vi "Power Accuracy Execute Measurement.vi"(0 "Plots":T11, 1 "Measurement Data In":T10[](array[typedef]), 2 "TestSetDef":T1={"General"={"ID"=0, "Model"="", "Dual Port?"=FALSE, "Options"="", "Options"={"E"=FALSE, "K"=FALSE, "H"=FALSE, "W"=FALSE, "F"=FALSE}, "Cal File"=path ""}, "Receiver"={"Fstart, MHz"=0.0, "Fstop MHz"=0.0, "Fstep MHz"=0.0, "IF, MHz"=0.0}, "RX Band"={"Fstart, MHz"=0.0, "Fstop MHz"=0.0}, "TX 1"={"Fstart, MHz"=0.0, "Fstop MHz"=0.0, "Pmax, dBm"=0.0, "Pstep, dB"=0.0}, "TX 2"={"Fstart, MHz"=0.0, "Fstop MHz"=0.0, "Pmax, dBm"=0.0, "Pstep, dB"=0.0}, "Low-side?"=TRUE}, 3 "Queue":refnum<queue>, 5 "Test Parameters":T2={"Stimulus"={"Power Start"=38, "Power Stop"=46, "Frequency Type"=enum."Band Edges", "Frequency Points"=[], "TX 1 Frequency (MHz)"={"Min"=0.0, "Max"=0.0}, "TX 2 Frequency (MHz)"={"Min"=0.0, "Max"=0.0}, "RX Frequency (MHz)"={"Min"=0.0, "Max"=0.0}, "Pad Model Number"="", "Pad Serial Number"="", "Pad Values"=[]}, "Measurement"={"DUT Port"=enum."Port 1", "Direction"=0}, "Display"={"Power"={"Min"=0, "Max"=0}, "Tolerance"={"Min"=0.0, "Max"=0.0}}, "Limit"={"Tolerance"=0.35}, "Calibration"={"Calibrated?"=FALSE}} {"Measurement"."Direction" items=["Reverse", "Forward", "Auxiliary"]}, 9 "Calculated Values":refnum<vi>, 11 "error in (no error)":errorcluster, 12 "Driver Refs In":T14, 13 "Measurements":refnum<vi>) -> (4 "Pass/Fail":bool[](array[boolean]), 6 "Test Parameters Out":T2={"Stimulus"={"Power Start"=38, "Power Stop"=46, "Frequency Type"=enum."Band Edges", "Frequency Points"=[], "TX 1 Frequency (MHz)"={"Min"=0.0, "Max"=0.0}, "TX 2 Frequency (MHz)"={"Min"=0.0, "Max"=0.0}, "RX Frequency (MHz)"={"Min"=0.0, "Max"=0.0}, "Pad Model Number"="", "Pad Serial Number"="", "Pad Values"=[]}, "Measurement"={"DUT Port"=enum."Port 1", "Direction"=0}, "Display"={"Power"={"Min"=0, "Max"=0}, "Tolerance"={"Min"=0.0, "Max"=0.0}}, "Limit"={"Tolerance"=0.35}, "Calibration"={"Calibrated?"=FALSE}} {"Measurement"."Direction" items=["Reverse", "Forward", "Auxiliary"]}, 10 "Measurement Data Out":T10[](array[typedef]), 14 "Driver Refs Out":T14, 15 "error out":errorcluster)   [LabVIEW 2011]
uses:
  TypeDefs/Power Accuracy Test Parameters.ctl
  TypeDefs/Power Accuracy Stimulus Parameters.ctl
  TypeDefs/Power Accuracy Measurement Parameters.ctl
  BPIMCore EXT/HW IO/DUTport.ctl
  BPIMCore EXT/HW IO/MeasMode.ctl
  TypeDefs/Power Accuracy Display Parameters.ctl
  TypeDefs/Power Accuracy Limit Parameters.ctl
  TypeDefs/Power Accuracy Calibration State.ctl
  drivers/PIM/PIM Driver Ref.ctl
  drivers/PWM/PWM Driver Ref.ctl
  TypeDefs/Power Accuracy Measurement Data.ctl
  TypeDefs/Power Accuracy Queue Cluster.ctl
  BPIMCore EXT/HW IO/Test Set Definition.ctl
  drivers/PIM/PIM Command.ctl
  drivers/PWM/PWM Parameters.ctl
  drivers/PWM/PWM Command.ctl
  Summitek EXT/Miscellaneous/OGAB Version.ctl
  <vilib>/Analysis/NI_AALBase.lvlib
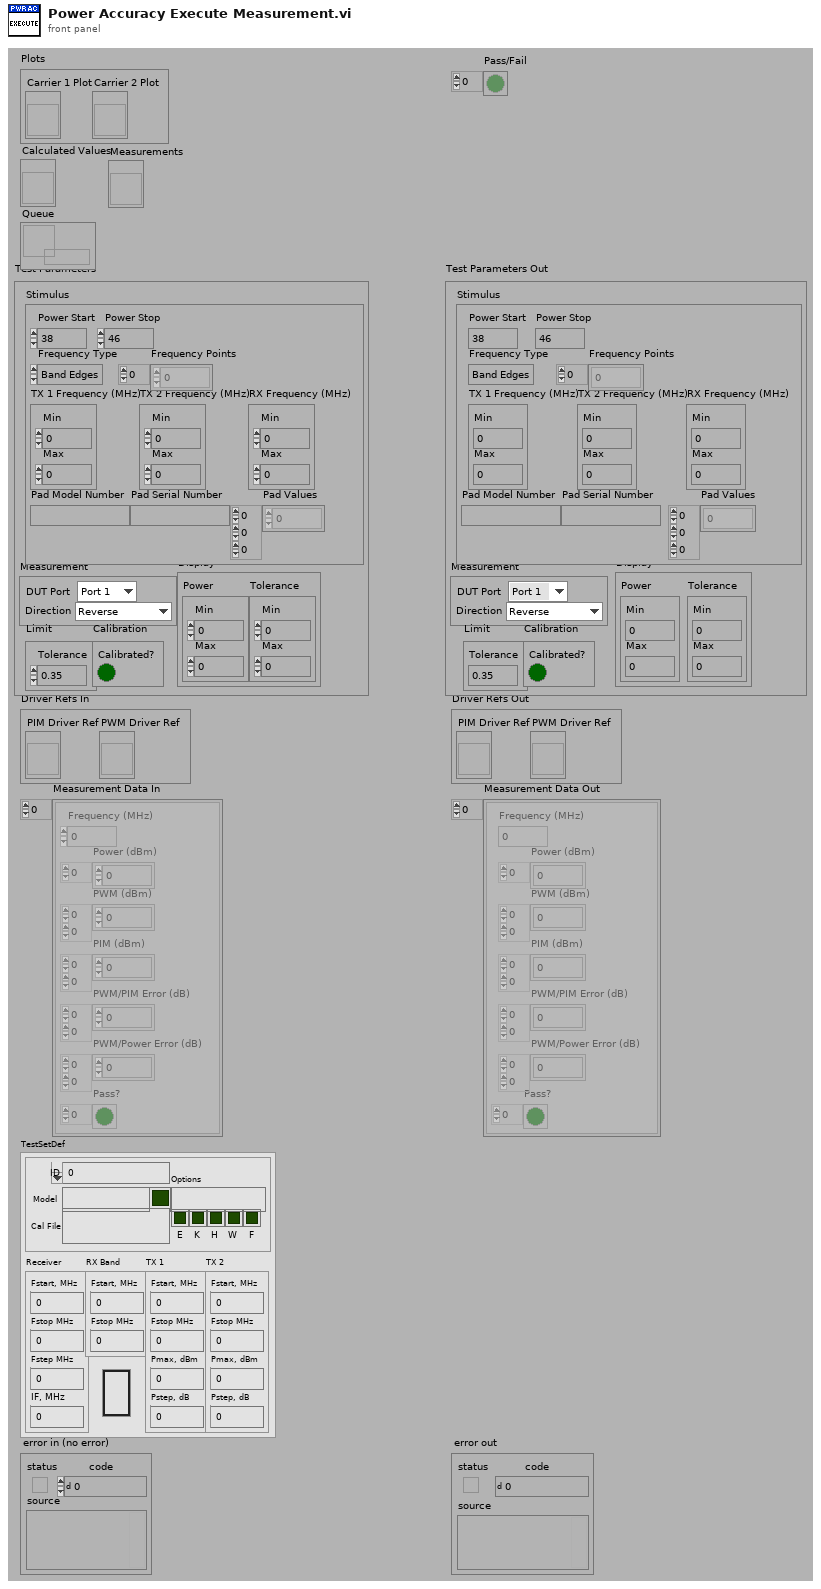
[diagram p1: front panel]
types:
  T1 = typedef "Test Set Definition.ctl" = cluster{"General":cluster{"ID":u32, "Model":string, "Dual Port?":bool, "Options":string, "Options":cluster{"E":bool, "K":bool, "H":bool, "W":bool, "F":bool}, "Cal File":path}, "Receiver":cluster{"Fstart, MHz":dbl, "Fstop MHz":dbl, "Fstep MHz":dbl, "IF, MHz":dbl}, "RX Band":cluster{"Fstart, MHz":dbl, "Fstop MHz":dbl}, "TX 1":cluster{"Fstart, MHz":dbl, "Fstop MHz":dbl, "Pmax, dBm":dbl, "Pstep, dB":dbl}, "TX 2":cluster{"Fstart, MHz":dbl, "Fstop MHz":dbl, "Pmax, dBm":dbl, "Pstep, dB":dbl}, "Low-side?":bool}
  T2 = typedef "Power Accuracy Test Parameters.ctl" = cluster{"Stimulus":T3, "Measurement":T4, "Display":T7, "Limit":T8, "Calibration":T9}
  T3 = typedef "Power Accuracy Stimulus Parameters.ctl" = cluster{"Power Start":i32, "Power Stop":i32, "Frequency Type":enum16{"Band Edges", "Custom"}, "Frequency Points":dbl[], "TX 1 Frequency (MHz)":cluster{"Min":dbl, "Max":dbl}, "TX 2 Frequency (MHz)":cluster{"Min":dbl, "Max":dbl}, "RX Frequency (MHz)":cluster{"Min":dbl, "Max":dbl}, "Pad Model Number":string, "Pad Serial Number":string, "Pad Values":dbl[][][]}
  T4 = typedef "Power Accuracy Measurement Parameters.ctl" = cluster{"DUT Port":T5, "Direction":T6}
  T5 = typedef "DUTport.ctl" = enum16{"Port 1", "Port 2"}
  T6 = typedef "MeasMode.ctl" = u16
  T7 = typedef "Power Accuracy Display Parameters.ctl" = cluster{"Power":cluster{"Min":i32, "Max":i32}, "Tolerance":cluster{"Min":dbl, "Max":dbl}}
  T8 = typedef "Power Accuracy Limit Parameters.ctl" = cluster{"Tolerance":dbl}
  T9 = typedef "Power Accuracy Calibration State.ctl" = cluster{"Calibrated?":bool}
  T10 = typedef "Power Accuracy Measurement Data.ctl" = cluster{"Frequency (MHz)":dbl, "Power (dBm)":i32[], "PWM (dBm)":dbl[][], "PIM (dBm)":dbl[][], "PWM/PIM Error (dB)":dbl[][], "PWM/Power Error (dB)":dbl[][], "Pass?":bool[]}
  T11 = cluster{"Carrier 1 Plot":refnum<vi>, "Carrier 2 Plot":refnum<vi>}
  T12 = typedef "PIM Driver Ref.ctl" = refnum<vi>
  T13 = typedef "PWM Driver Ref.ctl" = refnum<vi>
  T14 = cluster{"PIM Driver Ref":T12, "PWM Driver Ref":T13}
  T15 = typedef "PIM Stimulus.ctl" = cluster{"Carrier Frequencies":cluster{"C1 Freq, MHz":dbl, "C2 Freq, MHz":dbl}, "Carrier Powers":cluster{"C1 Power,dBm":dbl, "C2 Power, dBm":dbl}, "Measurement Parameters":T16, "Measurement Setup":cluster{"Meas Type":enum32{"Time", "Frequency"}, "TXStep":T20}}
  T16 = typedef "PIM Cmd Params.ctl" = cluster{"IM Order":T17, "Averaging":T18, "Direction":T6, "Enable ALC?":bool, "Enable SingleIM?":bool, "Display Units":T19, "VA Hold?":bool, "DUT PORT":T5}
  T17 = typedef "IMOrder.ctl" = u8
  T18 = typedef "HW Averaging.ctl" = u16
  T19 = typedef "display_unit_format.ctl" = enum16{"dBm", "dBc"}
  T20 = typedef "PIM Sweep Step Size.ctl" = u16
  T21 = typedef "PIM Command.ctl" = enum16{"LOAD", "KEEP ALIVE", "VALIDATE", "INITIALIZE", "PRESET", "GET CALIBRATION", "SET STIMULUS", "TOGGLE TX POWER", "SET TX ON", "SET TX OFF", "MEASURE", "UNLOAD"}
  T22 = typedef "PWM Parameters.ctl" = cluster{"Zero":bool, "Blank Screen":bool, "Offset":bool, "Offset Value":dbl, "Frequency (MHz)":dbl}
  T23 = typedef "PWM Command.ctl" = enum16{"LOAD", "INITIALIZE", "PRESET", "GET STIMULUS", "SET STIMULUS", "MEASURE", "RELEASE", "UNLOAD", "GET CALIBRATION", "CALIBRATE"}
  T24 = typedef "OGAB Version.ctl" = cluster{"Version":string, "Build Number":u32, "Build Date/Time":dbl}
  T25 = typedef "Power Accuracy Queue Cluster.ctl" = cluster{"Command":string, "Test Parameters":T2}
  T26 = typedef "PIM Results.ctl" = cluster{"TxFreqs":dbl[], "TxPower":dbl[], "TxOn":bool[], "IMPower(s)":dbl[], "IMFreq(s)":dbl[], "Tx Stat":cluster{"CheckTx 1":bool, "Unlev Tx 1":bool, "Sql Tx 1":bool, "CheckTx 2":bool, "Unlev Tx 2":bool, "Sql Tx 2":bool}, "IM Overload":bool, "IMPower_dBc(s)":dbl[]}
  T27 = typedef "PWM Measurement.ctl" = dbl
  T28 = cluster{"duplicate driver ref":T12, "PWM Driver Ref":T13}
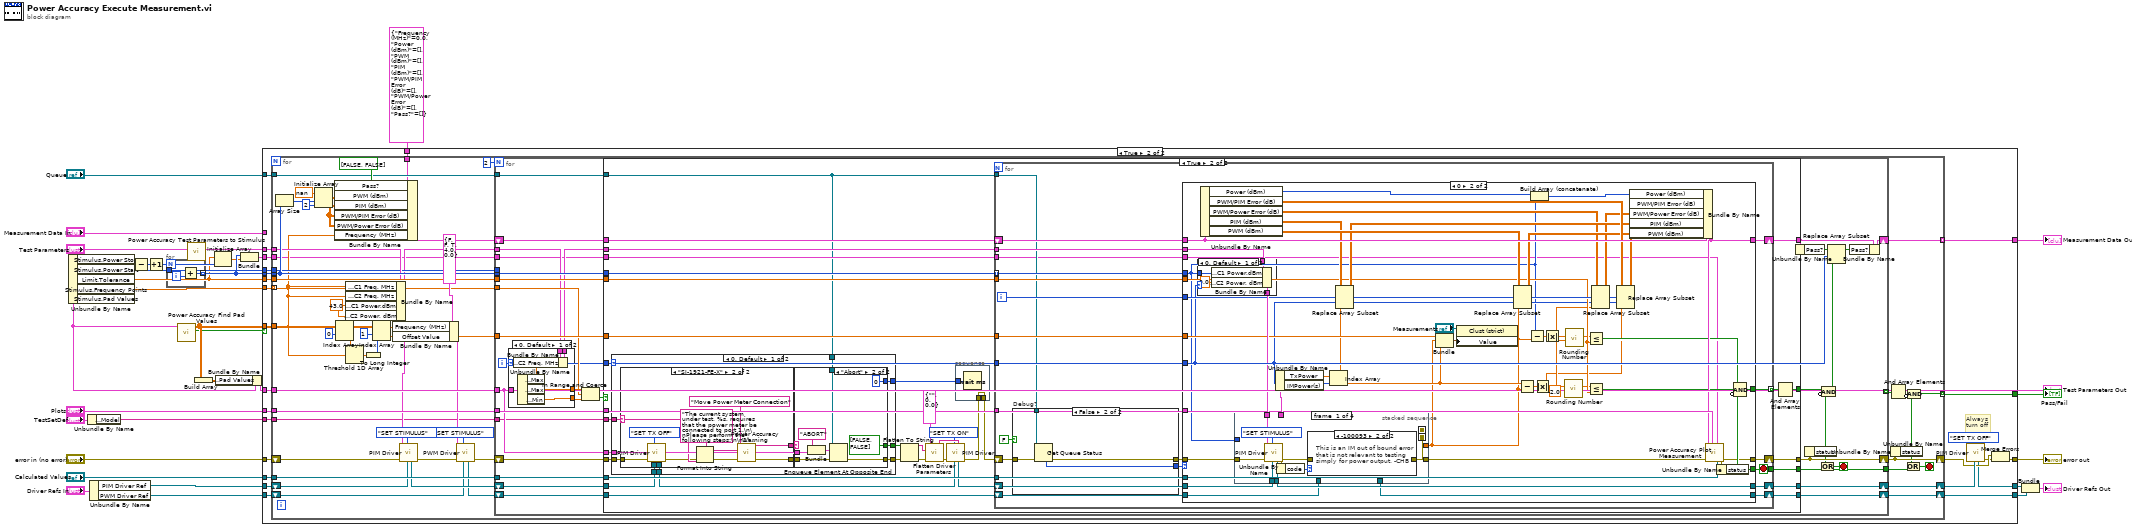
[diagram p0: block diagram]
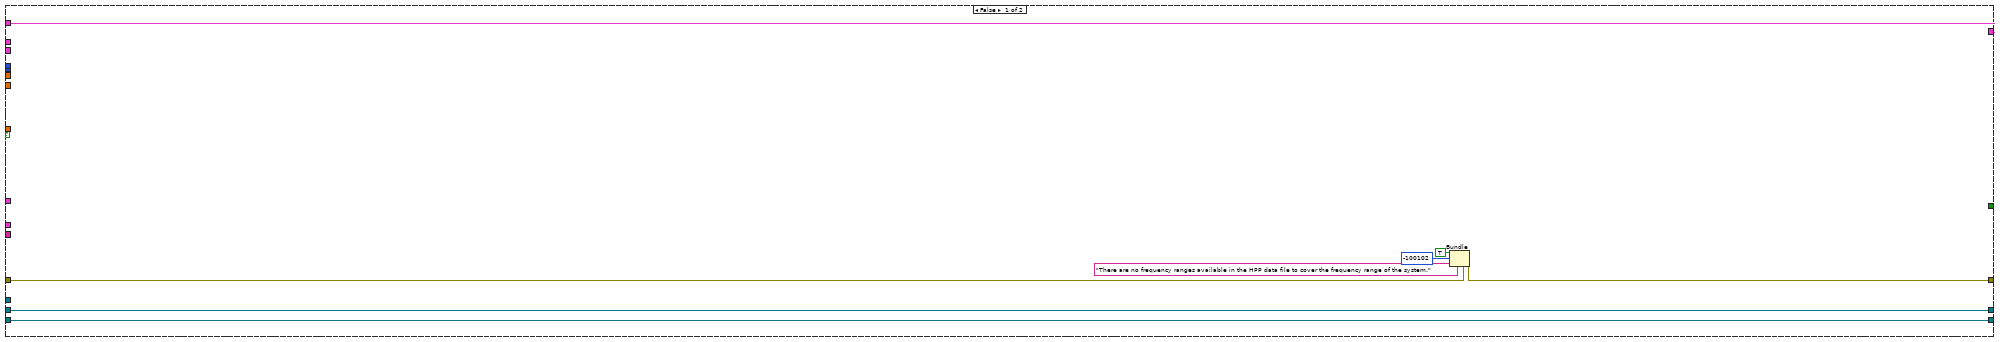
[diagram p2: hidden frame]
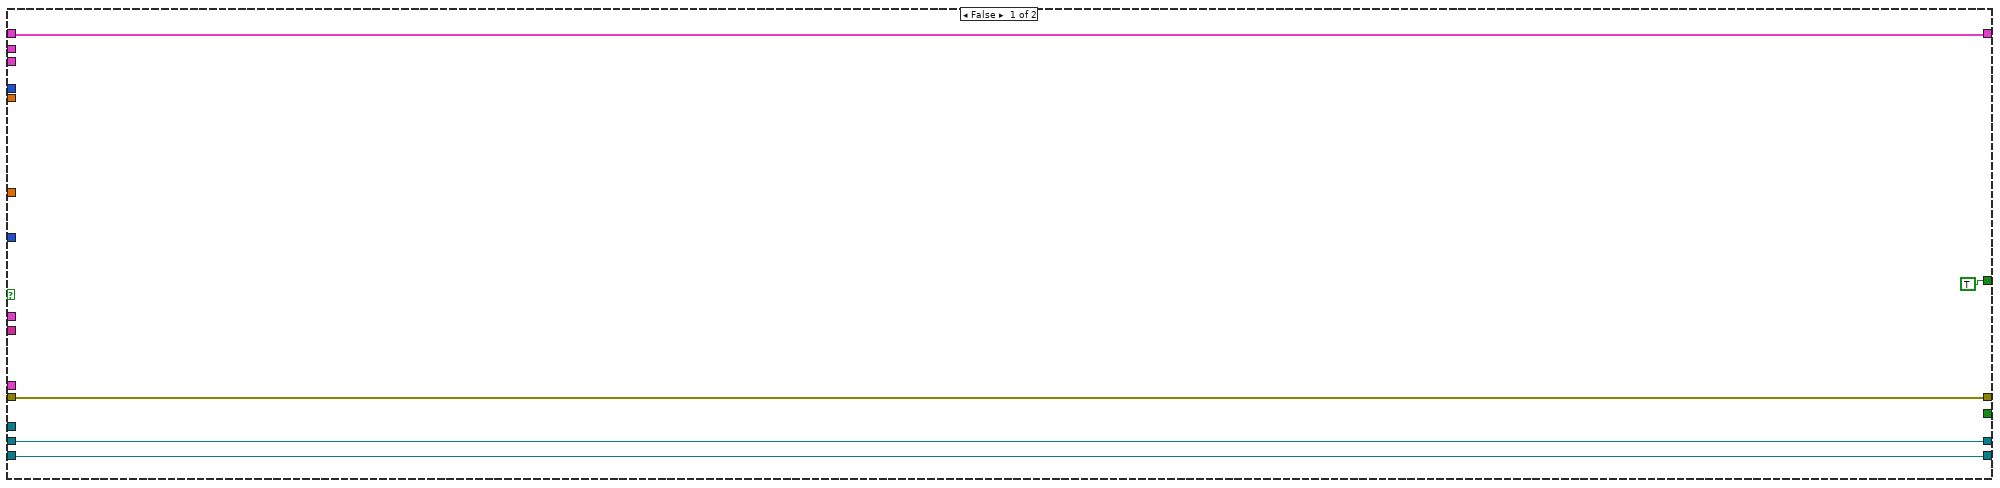
[diagram p3: hidden frame]
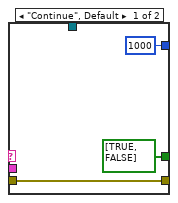
[diagram p4: hidden frame]
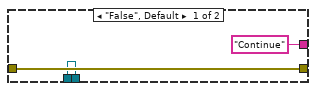
[diagram p5: hidden frame]
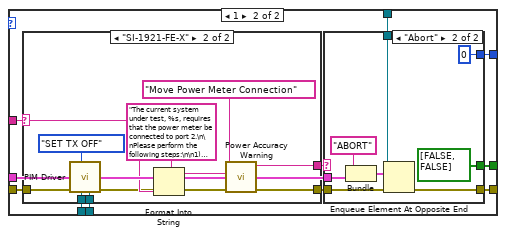
[diagram p6: hidden frame]
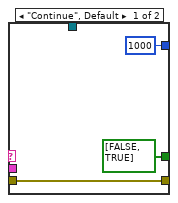
[diagram p7: hidden frame]
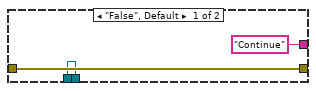
[diagram p8: hidden frame]
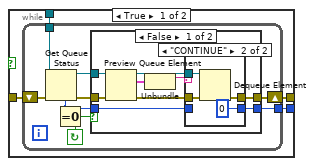
[diagram p9: hidden frame]
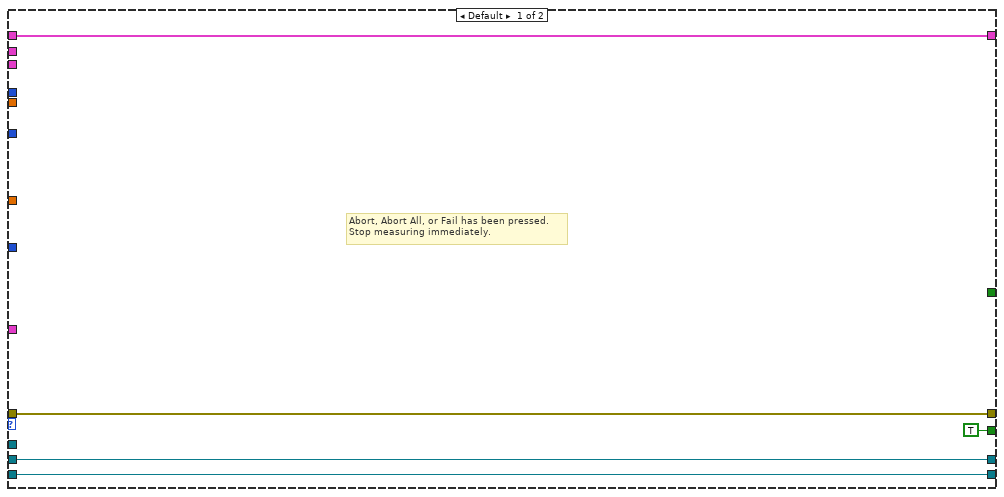
[diagram p12: hidden frame]
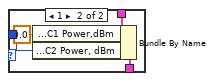
[diagram p13: hidden frame]
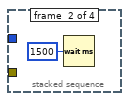
[diagram p15: hidden frame]
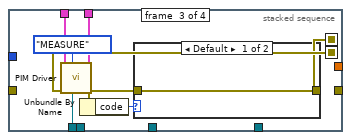
[diagram p16: hidden frame]
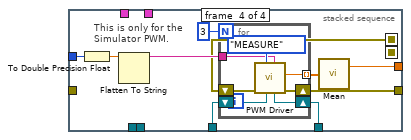
[diagram p18: hidden frame]
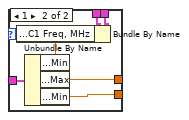
[diagram p19: hidden frame]
diagram:
  n1 = Unbundle By Name("Test Parameters") -> ("Stimulus.Power Stop"=w31:i32, "Stimulus.Power Start"=w30:i32, "Limit.Tolerance"=w10:dbl, "Stimulus.Frequency Points"=w23:dbl[])  [unwired: 1 out]
  n2 = Unbundle By Name("TestSetDef") -> ("General.Model"=w1:string)
  n3 = Unbundle By Name("Driver Refs In") -> ("PIM Driver Ref"=w25:T12, "PWM Driver Ref"=w26:T13)
  n4 = Subtract(x=w31, y=w30) -> (x-y=w32:i32)
  n5 = Increment(x=w32) -> (x+1=w11:i32)
  n6 = for {
    N: w11 -> [_]
    tunnel: w30 -> [w35]
    tunnel: [w33] -> w12 mode=indexing
    i -> [w34]
    n7 = Add(x=w35, y=w34) -> (x+y=w33:i32)
  }
  n8 = call "Power Accuracy Find Pad Values.vi"("Test Parameters"="Test Parameters") -> ("Values Present?"=w3:bool, "Pad Values Out"=w5:dbl[][])  [unwired: 9 in]
  n9 = call "Power Accuracy Test Parameters to Stimulus.vi"("Power Accuracy Test Parameters"="Test Parameters") -> ("PIM Measurement Stimulus"=w28:T15)  [unwired: 10 out]
  n10 = Build Array(w5) -> (w15:dbl[][][])
  n11 = Initialize Array(w10, w11) -> (w9:dbl[])
  n12 = Bundle By Name(cluster="Test Parameters", "Stimulus.Pad Values"=w15) -> (w14:T2)
  "Test Parameters Out" <- w14
  n13 = Bundle(w12, w9) -> (w8:cluster{i32[], dbl[]})  [unwired: 1 in]
  n14 = case shown="True" w3 {
    tunnel: w10 -> [_ w68]
    tunnel: w12 -> [_ w67]
    tunnel: w30 -> [_ w66]
    tunnel: w28 -> [_ w65]
    tunnel: T10 {"Frequency (MHz)"=0.0, "Power (dBm)"=[], "PWM (dBm)"=[], "PIM (dBm)"=[], "PWM/PIM Error (dB)"=[], "PWM/Power Error (dB)"=[], "Pass?"=[]} ("Measurement Data In") -> [_ w45]
    tunnel: [w41 w64] -> w16
    tunnel: [w36 w63] -> w27
    tunnel: w26 -> [w42 w60]
    tunnel: w25 -> [w43 w59]
    tunnel: "Plots" -> [_ w58]
    tunnel: "error in (no error)" -> [w37 w57]
    tunnel: w23 -> [_ w56]
    tunnel: w5 -> [_ w55]
    tunnel: [w43 w54] -> w21
    tunnel: [w42 w53] -> w20
    tunnel: "Measurement Data In" -> [w41 _]
    tunnel: w14 -> [_ w50]
    tunnel: "Calculated Values" -> [_ w49]
    tunnel: [_ w48] -> w17
    tunnel: "Queue" -> [_ w47]
    tunnel: w8 -> [_ w46]
    tunnel: w1 -> [_ w44]
    frame False {
      n15 = Bundle(cluster=w37, "status"=TRUE, "code"=-100102, "source"="There are no frequency ranges available in the HPP data file to cover the frequency range of the system.") -> (w36:errorcluster)
    }
    frame True {
      # "Always\nturn off"
      n16 = for {
        tunnel: w68 -> [w117]
        tunnel: w58 -> [w116]
        tunnel: w56 -> [w72] mode=indexing
        tunnel: w67 -> [w110]
        tunnel: w66 -> [w82]
        tunnel: w65 -> [w87]
        tunnel: w55 -> [w96]
        tunnel: w45 -> [w92]
        tunnel: [w109] -> w64 mode=indexing
        tunnel: [w101] -> w48 mode=indexing
        shift-right: [w107] -> w61
        shift-left: w57 -> [w85]
        shift-right: [w114] -> w62
        shift-left: w59 -> [w84]
        shift-right: [w115] -> w53
        shift-left: w60 -> [w77]
        tunnel: w50 -> [w103]
        tunnel: w49 -> [w102]
        tunnel: w47 -> [w94]
        tunnel: w46 -> [w70]
        tunnel: w44 -> [w69]
        stop <- w88 stop-if-true
        w73 = 43.0 ("Carrier Powers.C1 Power,dBm")
        n17 = Array Size(array=w110) -> (size(s)=w112:i32)
        n18 = Initialize Array(nan ("Power (dBm)"), w112, 2 ("dimension size")) -> (w91:dbl[][])
        n19 = Bundle By Name(cluster=w92, "Pass?"=bool[] [FALSE, FALSE], "PWM (dBm)"=w91, "PIM (dBm)"=w91, "PWM/PIM Error (dB)"=w91, "PWM/Power Error (dB)"=w91, "Frequency (MHz)"=w72) -> (w93:T10)
        n20 = Index Array(array=w96, index (row)=0 ("disabled index (col)")) -> (element=w95:dbl[])  [unwired: 1 in]
        n21 = Threshold 1D Array(2:w72, 3:w95) -> (0:w106:dbl)  [unwired: 1 out]
        n22 = Bundle By Name(cluster=w87, "Carrier Frequencies.C1 Freq, MHz"=w72, "Carrier Frequencies.C2 Freq, MHz"=w72, "Carrier Powers.C1 Power,dBm"=w73, "Carrier Powers.C2 Power, dBm"=w73) -> (w81:T15)
        n23 = To Long Integer(number=w106) -> (32bit integer=w104:i32)
        n24 = Index Array(array=w96, index (row)=1 ("disabled index (col)"), index (col)=w104) -> (element=w74:dbl)
        n25 = Bundle By Name(cluster=T22 {"Zero"=FALSE, "Blank Screen"=FALSE, "Offset"=TRUE, "Offset Value"=4.0, "Frequency (MHz)"=0.0} ("PWM Stimulus"), "Frequency (MHz)"=w72, "Offset Value"=w74) -> (w71:T22)
        n26 = call "PIM Driver.vi"("Driver Ref (null)"=w84, "PIM Command"=PIM_Command."SET STIMULUS", "error in (no error)"=w85, "Stimulus"=w81) -> ("error out"=w78:errorcluster, "duplicate driver ref"=w83:T12)  [unwired: 1 in, 5 out]
        n27 = call "PWM Driver.vi"("Drv Refnum"=w77, "PWM Command"=PWM_Command."SET STIMULUS", "error in (no error)"=w78, "PWM Stimulus"=w71) -> ("error out"=w75:errorcluster, "dup Drv Refnum"=w76:T13)  [unwired: 4 in, 2 out]
        n28 = for {
          N: 2 -> [_]
          tunnel: w117 -> [w149]
          tunnel: w81 -> [w125]
          tunnel: w116 -> [w148]
          shift-right: [w141] -> w107
          shift-left: w75 -> [w120]
          tunnel: w110 -> [w145]
          tunnel: w82 -> [_]
          shift-right: [w144] -> w114
          shift-left: w83 -> [w121]
          shift-right: [w146] -> w115
          shift-left: w76 -> [w147]
          tunnel: [w135] -> w100 mode=indexing
          shift-right: [w133] -> w109
          shift-left: w93 -> [w140]
          tunnel: w74 -> [w139]
          tunnel: w103 -> [w119]
          tunnel: w102 -> [w138]
          tunnel: w94 -> [w122]
          tunnel: [w128] -> w89
          tunnel: w72 -> [w127]
          tunnel: w70 -> [w123]
          tunnel: w69 -> [w118]
          i -> [w126]
          stop <- w129 stop-if-true
          n29 = case shown="0, Default" w126 {
            tunnel: [w420 w426] -> w143
            tunnel: [w419 w425] -> w142
            tunnel: w119 -> [w415 w421]
            tunnel: w125 -> [w417 w423]
            tunnel: [w416 w422] -> w124
            frame 0, Default {
              n30 = Unbundle By Name(w415) -> ("Stimulus.TX 2 Frequency (MHz).Max"=w418:dbl, "Stimulus.TX 1 Frequency (MHz).Max"=w420:dbl, "Stimulus.TX 1 Frequency (MHz).Min"=w419:dbl)
              n31 = Bundle By Name(cluster=w417, "Carrier Frequencies.C2 Freq, MHz"=w418) -> (w416:T15)
            }
            frame 1 {
              n32 = Unbundle By Name(w421) -> ("Stimulus.TX 1 Frequency (MHz).Min"=w424:dbl, "Stimulus.TX 2 Frequency (MHz).Max"=w426:dbl, "Stimulus.TX 2 Frequency (MHz).Min"=w425:dbl)
              n33 = Bundle By Name(cluster=w423, "Carrier Frequencies.C1 Freq, MHz"=w424) -> (w422:T15)
            }
          }
          n34 = In Range and Coerce(upper limit=w143, x=w127, lower limit=w142) -> (In Range?=w132:bool)  [unwired: 1 out]
          n35 = case shown="True" w132 {
            tunnel: w149 -> [_ w189]
            tunnel: w148 -> [_ w188]
            tunnel: w147 -> [w152 w187]
            tunnel: [w152 w186] -> w146
            tunnel: w121 -> [w153 w162]
            tunnel: w124 -> [_ w185]
            tunnel: w145 -> [_ w184]
            tunnel: [w153 w183] -> w144
            tunnel: [w154 w182] -> w141
            tunnel: w120 -> [w154 w163]
            tunnel: w140 -> [w150 w181]
            tunnel: w139 -> [_ w180]
            tunnel: w138 -> [_ w179]
            tunnel: w126 -> [_ w164]
            tunnel: [w150 w178] -> w134
            tunnel: [TRUE w176] -> w131
            tunnel: w122 -> [_ w158]
            tunnel: [_ w175] -> w128
            tunnel: w123 -> [_ w165]
            tunnel: w119 -> [_ w157]
            tunnel: w118 -> [_ w155]
            frame False {
            }
            frame True {
              n36 = case shown="0, Default" w164 {
                tunnel: w163 -> [w200 w236]
                tunnel: w162 -> [w199 w229]
                tunnel: [w198 w228] -> w161
                tunnel: [w197 w232] -> w160
                tunnel: [w196 w231] -> w159
                tunnel: w158 -> [w194 w233]
                tunnel: w157 -> [w192 w235]
                tunnel: [w191 w227] -> w156
                tunnel: w155 -> [w190 w226]
                frame 0, Default {
                  n37 = case shown="\"SI-1921-FE-X\"" w190 {
                    selector: w190 -> [_ w221]
                    tunnel: w200 -> [w214 w218]
                    tunnel: [w214 w224] -> w195
                    tunnel: ["Continue" ("Dialog Response") w220] -> w193
                    tunnel: w199 -> [w212 w216]
                    tunnel: [w212 w215] -> w198
                    frame "False", Default {
                    }
                    frame "SI-1921-FE-X" {
                      n38 = call "PIM Driver.vi"("Driver Ref (null)"=w216, "PIM Command"=PIM_Command."SET TX OFF", "error in (no error)"=w218) -> ("error out"=w217:errorcluster, "duplicate driver ref"=w215:T12)  [unwired: 2 in, 5 out]
                      n39 = Format Into String(format string="The current system under test, %s, requires that the power meter be connected to port 1.\n\nPlease perform the following steps:\n\n1)  Connect the Power Sensor to port 1;\n2)  Press Continue." ("F button name (\"Cancel\")"), w221) -> (resulting string=w222:string)  [unwired: 2 in, 1 out]
                      n40 = call "Power Accuracy Warning.vi"("error in (no error)"=w217, "Message"=w222, "Header"="Move Power Meter Connection" ("F button name (\"Cancel\")")) -> ("error out"=w224:errorcluster, "Dialog Response"=w220:string)  [unwired: 7 in]
                    }
                  }
                  n41 = case shown="\"Abort\"" w193 {
                    tunnel: [bool[] [TRUE, FALSE] bool[] [FALSE, FALSE]] -> w196
                    tunnel: [u32 1000 ("milliseconds to wait") u32 0 ("milliseconds to wait")] -> w197
                    tunnel: w195 -> [w201 w209]
                    tunnel: [w201 w208] -> w191
                    tunnel: w194 -> [_ w205]
                    tunnel: w192 -> [_ w204]
                    frame "Continue", Default {
                    }
                    frame "Abort" {
                      n42 = Bundle("ABORT", "Test Parameters"=w204) -> (w206:cluster{string, "Test Parameters":T2})  [unwired: 1 out]
                      n43 = Enqueue Element At Opposite End(queue=w205, element=w206, error in (no error)=w209) -> (error out=w208:errorcluster)  [unwired: 1 in, 2 out]
                    }
                  }
                }
                frame 1 {
                  n44 = case shown="\"SI-1921-FE-X\"" w226 {
                    selector: w226 -> [_ w257]
                    tunnel: w236 -> [w250 w254]
                    tunnel: [w250 w260] -> w230
                    tunnel: ["Continue" ("Dialog Response") w256] -> w234
                    tunnel: w229 -> [w248 w252]
                    tunnel: [w248 w251] -> w228
                    frame "False", Default {
                    }
                    frame "SI-1921-FE-X" {
                      n45 = call "PIM Driver.vi"("Driver Ref (null)"=w252, "PIM Command"=PIM_Command."SET TX OFF", "error in (no error)"=w254) -> ("error out"=w253:errorcluster, "duplicate driver ref"=w251:T12)  [unwired: 2 in, 5 out]
                      n46 = Format Into String(format string="The current system under test, %s, requires that the power meter be connected to port 2.\n\nPlease perform the following steps:\n\n1)  Connect the Power Sensor to port 2;\n2)  Press Continue." ("F button name (\"Cancel\")"), w257) -> (resulting string=w258:string)  [unwired: 2 in, 1 out]
                      n47 = call "Power Accuracy Warning.vi"("error in (no error)"=w253, "Message"=w258, "Header"="Move Power Meter Connection" ("F button name (\"Cancel\")")) -> ("error out"=w260:errorcluster, "Dialog Response"=w256:string)  [unwired: 7 in]
                    }
                  }
                  n48 = case shown="\"Abort\"" w234 {
                    tunnel: [bool[] [FALSE, TRUE] bool[] [FALSE, FALSE]] -> w231
                    tunnel: [u32 1000 ("milliseconds to wait") u32 0 ("milliseconds to wait")] -> w232
                    tunnel: w230 -> [w237 w245]
                    tunnel: [w237 w244] -> w227
                    tunnel: w233 -> [_ w241]
                    tunnel: w235 -> [_ w240]
                    frame "Continue", Default {
                    }
                    frame "Abort" {
                      n49 = Bundle("ABORT", "Test Parameters"=w240) -> (w242:cluster{string, "Test Parameters":T2})  [unwired: 1 out]
                      n50 = Enqueue Element At Opposite End(queue=w241, element=w242, error in (no error)=w245) -> (error out=w244:errorcluster)  [unwired: 1 in, 2 out]
                    }
                  }
                }
              }
              n51 = Flatten To String(anything=w159, error in (no error)=w156) -> (data string=w170:string, error out=w173:errorcluster)  [unwired: 2 in, 1 out]
              n52 = call "Flatten Driver Parameters.vi"("error in (no error)"=w173, "Flattened Driver Parameters (\"\")"=w170, "Driver Version"=T24 {"Version"="", "Build Number"=0, "Build Date/Time"=0.0}) -> ("error out"=w172:errorcluster, "Flattened Driver Parameters with Version"=w171:string)  [unwired: 3 in]
              n53 = call "PIM Driver.vi"("PIM Driver Name/Configuration"=w171, "Driver Ref (null)"=w161, "PIM Command"=PIM_Command."SET TX ON", "error in (no error)"=w172) -> ("error out"=w169:errorcluster, "duplicate driver ref"=w167:T12)  [unwired: 1 in, 5 out]
              n54 = stacked-sequence {
                tunnel: w169 -> [w263]
                tunnel: [w263] -> w166
                tunnel: w160 -> [w262]
                frame #0 {
                  n55 = Wait (ms)(milliseconds to wait=w262) -> ()  [unwired: 1 out]
                }
              }
              n56 = for {
                tunnel: w185 -> [w286]
                tunnel: [w271] -> w177 mode=indexing
                tunnel: w188 -> [w279]
                shift-right: [w273] -> w186
                shift-left: w187 -> [w285]
                shift-right: [w274] -> w183
                shift-left: w167 -> [w284]
                tunnel: w189 -> [w277]
                shift-right: [w278] -> w178
                shift-left: w181 -> [w282]
                shift-right: [w275] -> w182
                shift-left: w166 -> [w270]
                tunnel: w184 -> [w281] mode=indexing
                tunnel: w180 -> [w283]
                tunnel: w164 -> [w280]
                tunnel: w179 -> [w272]
                tunnel: w158 -> [w269]
                tunnel: [w268] -> w175
                tunnel: w165 -> [w267]
                i -> [w276]
                stop <- w268 stop-if-true
                n57 = case "Debug?" shown="False" FALSE {
                  tunnel: w270 -> [w290 w319]
                  tunnel: w269 -> [w289 w318]
                  tunnel: [w288 w317] -> w266
                  tunnel: [w287 w316] -> w265
                  frame True {
                    n58 = while {
                      tunnel: w289 -> [w297]
                      shift-right: [w294] -> w288
                      shift-left: w290 -> [w298]
                      tunnel: [w292] -> w287
                      stop <- w291 continue-if-true
                      n59 = Get Queue Status(queue=w297, error in (no error)=w298) -> (queue out=w295:refnum<queue>, error out=w296:errorcluster, # elements in queue=w293:i32)  [unwired: 1 in, 5 out]
                      n60 = Equal To 0?(x=w293) -> (x = 0?=w291:bool)
                      n61 = case shown="False" w291 {
                        tunnel: w296 -> [w307 w315]
                        tunnel: w295 -> [w306 _]
                        tunnel: [w302 w315] -> w294
                        tunnel: w293 -> [w300 w314]
                        tunnel: [w299 w314] -> w292
                        frame False {
                          n62 = Preview Queue Element(queue=w306, error in (no error)=w307) -> (queue out=w301:refnum<queue>, element=w305:T25, error out=w303:errorcluster)  [unwired: 1 in, 1 out]
                          n63 = Unbundle(w305) -> ("Command"=w304:string)  [unwired: 1 out]
                          n64 = case shown="\"CONTINUE\"" w304 {
                            tunnel: w303 -> [w309 w313]
                            tunnel: [w309 w312] -> w302
                            tunnel: w301 -> [_ w311]
                            tunnel: w300 -> [w308 _]
                            tunnel: [w308 0 ("# elements in queue")] -> w299
                            frame "False", Default {
                            }
                            frame "CONTINUE" {
                              n65 = Dequeue Element(queue=w311, error in (no error)=w313) -> (error out=w312:errorcluster)  [unwired: 1 in, 3 out]
                            }
                          }
                        }
                        frame True {
                        }
                      }
                    }
                  }
                  frame False {
                    n66 = Get Queue Status(queue=w318, error in (no error)=w319) -> (error out=w317:errorcluster, # elements in queue=w316:i32)  [unwired: 1 in, 6 out]
                  }
                }
                n67 = case shown="0" w265 {
                  tunnel: w286 -> [_ w370]
                  tunnel: w285 -> [w321 w334]
                  tunnel: [w322 w369] -> w274
                  tunnel: [w321 w336] -> w273
                  tunnel: w284 -> [w322 w365]
                  tunnel: w283 -> [_ w340]
                  tunnel: w266 -> [w323 w352]
                  tunnel: w282 -> [w324 w363]
                  tunnel: w281 -> [_ w333]
                  tunnel: w280 -> [_ w337]
                  tunnel: w279 -> [_ w354]
                  tunnel: [w324 w353] -> w278
                  tunnel: w277 -> [_ w343]
                  tunnel: [w323 w331] -> w275
                  tunnel: w276 -> [_ w345]
                  tunnel: w272 -> [_ w351]
                  tunnel: [_ w349] -> w271
                  tunnel: [TRUE ("status") w348] -> w268
                  tunnel: w267 -> [_ w332]
                  frame Default {
                    # "Abort, Abort All, or Fail has been pressed.\nStop measuring immediately."
                  }
                  frame 0 {
                    w327 = -2.0 ("Power of ten")
                    n68 = case shown="0, Default" w337 {
                      tunnel: w370 -> [w374 w378]
                      tunnel: [w373 w377] -> w366
                      tunnel: w333 -> [w372 w376]
                      frame 0, Default {
                        n69 = Bundle By Name(cluster=w374, "Carrier Powers.C1 Power,dBm"=w372, "Carrier Powers.C2 Power, dBm"=0.0) -> (w373:T15)
                      }
                      frame 1 {
                        n70 = Bundle By Name(cluster=w378, "Carrier Powers.C1 Power,dBm"=0.0, "Carrier Powers.C2 Power, dBm"=w376) -> (w377:T15)
                      }
                    }
                    n71 = Unbundle By Name(w363) -> ("Power (dBm)"=w361:i32[], "PWM/PIM Error (dB)"=w358:dbl[][], "PWM/Power Error (dB)"=w347:dbl[][], "PIM (dBm)"=w359:dbl[][], "PWM (dBm)"=w360:dbl[][])
                    n72 = stacked-sequence {
                      seq-local: [w380 _ _ _] -> [_ _ w391 _]
                      seq-local: [_ _ w390 _] -> [_ _ _ w398]
                      tunnel: [w385 _ _ _] -> w369
                      tunnel: [_ _ w389 _] -> w367
                      tunnel: w366 -> [w384 _ w393 _]
                      tunnel: w365 -> [w383 _ w394 _]
                      tunnel: w352 -> [w382 _ _ _]
                      tunnel: [_ _ _ w399] -> w335
                      tunnel: [_ _ _ w400] -> w336
                      tunnel: [_ _ _ w404] -> w330
                      tunnel: w334 -> [_ _ _ w406]
                      tunnel: w333 -> [_ _ _ w402]
                      frame #0 {
                        n73 = call "PIM Driver.vi"("Driver Ref (null)"=w383, "PIM Command"=PIM_Command."SET STIMULUS", "error in (no error)"=w382, "Stimulus"=w384) -> ("error out"=w381:errorcluster, "duplicate driver ref"=w385:T12)  [unwired: 1 in, 5 out]
                        n74 = Unbundle By Name(w381) -> ("code"=w379:i32)
                        n75 = case shown="-100093" w379 {
                          tunnel: w381 -> [w387 _]
                          tunnel: [w387 _] -> w380
                          frame Default {
                          }
                          frame -100093 {
                            # "This is an IM out of bound error\nthat is not relevant to testing\nsimply for power output. -CHB"
                          }
                        }
                      }
                      frame #1 {
                        n76 = Wait (ms)(milliseconds to wait=u32 1500) -> ()  [unwired: 1 out]
                      }
                      frame #2 {
                        n77 = call "PIM Driver.vi"("Driver Ref (null)"=w394, "PIM Command"=PIM_Command."MEASURE", "error in (no error)"=w391, "Stimulus"=w393) -> ("error out"=w392:errorcluster, "Measurement Results"=w389:T26)  [unwired: 1 in, 5 out]
                        n78 = Unbundle By Name(w392) -> ("code"=w396:i32)
                        n79 = case shown="Default" w396 {
                          tunnel: w392 -> [w397 _]
                          tunnel: [w397 _] -> w390
                          frame Default {
                          }
                          frame -100093 {
                            # "This is an IM out of bound error\nthat is not relevant to testing\nsimply for power output. -CHB"
                          }
                        }
                      }
                      frame #3 {
                        # "This is only for the\nSimulator PWM."
                        n80 = To Double Precision Float(number=w402) -> (double precision float=w401:dbl)
                        n81 = Flatten To String(anything=w401) -> (data string=w403:string)  [unwired: 3 in, 2 out]
                        n82 = for {
                          N: 3 -> [_]
                          tunnel: [w411] -> w405 mode=indexing
                          shift-right: [w413] -> w399
                          shift-left: w398 -> [w412]
                          tunnel: w403 -> [w409]
                          shift-right: [w408] -> w400
                          shift-left: w406 -> [w410]
                          n83 = call "PWM Driver.vi"("PWM Configuration (\"\")"=w409, "Drv Refnum"=w410, "PWM Command"=PWM_Command."MEASURE", "error in (no error)"=w412) -> ("error out"=w413:errorcluster, "PWM Measurement"=w411:T27, "dup Drv Refnum"=w408:T13)  [unwired: 4 in, 1 out]
                        }
                        n84 = call <vilib>:"Mean.vi"("X"=w405) -> ("mean"=w404:dbl)  [unwired: 1 out]
                      }
                    }
                    n85 = Unbundle By Name(w367) -> ("TxPower"=w368:dbl[])  [unwired: 1 out]
                    n86 = Index Array(array=w368, index=w337) -> (element=w338:dbl)
                    n87 = Replace Array Subset(array=w359, new element=w338, index (row)=w345, index (col)=w337) -> (w356:dbl[][])
                    n88 = Bundle("Numeric"=w340, "mean"=w330, w338) -> (w339:cluster{"Numeric":dbl, "mean":dbl, dbl})  [unwired: 1 in]
                    n89 = property class="Clust (strict)"(reference="Measurements", "Value"=w339) -> ()  [unwired: 1 in, 2 out]
                    n90 = Replace Array Subset(array=w360, new element=w330, index (row)=w345, index (col)=w337) -> (w357:dbl[][])
                    n91 = Subtract(x=w338, y=w330) -> (x-y=w364:dbl)
                    n92 = Subtract(x=w333, y=w330) -> (x-y=w344:dbl)
                    n93 = Build Array (concatenate)(w361, w333) -> (w362:i32[])
                    n94 = Absolute Value(x=w364) -> (abs(x)=w325:dbl)
                    n95 = Absolute Value(x=w344) -> (abs(x)=w326:dbl)
                    n96 = call "Rounding Number.vi"("Power of ten"=w327, "Number to round"=w325) -> ("Rounded number"=w328:dbl)  [unwired: 8 in, 1 out]
                    n97 = call "Rounding Number.vi"("Power of ten"=w327, "Number to round"=w326) -> ("Rounded number"=w329:dbl)  [unwired: 8 in, 1 out]
                    n98 = Less Or Equal?(x=w329, y=w343) -> (x <= y?=w342:bool)
                    n99 = Less Or Equal?(x=w328, y=w343) -> (x <= y?=w350:bool)
                    n100 = Replace Array Subset(array=w347, new element=w326, index (row)=w345, index (col)=w337) -> (w346:dbl[][])
                    n101 = Replace Array Subset(array=w358, new element=w325, index (row)=w345, index (col)=w337) -> (w355:dbl[][])
                    n102 = Bundle By Name(cluster=w363, "Power (dBm)"=w362, "PWM/PIM Error (dB)"=w355, "PWM/Power Error (dB)"=w346, "PIM (dBm)"=w356, "PWM (dBm)"=w357) -> (w353:T10)
                    n103 = call "Power Accuracy Plot Measurement.vi"("Calculated Values"=w351, "Tolerance (dBm)"=w332, "Plots"=w354, "error in (no error)"=w335, "Measurement Data"=w353) -> ("error out"=w331:errorcluster)  [unwired: 6 in]
                    n104 = Unbundle By Name(w331) -> ("status"=w348:bool)
                    n105 = Compound Arithmetic op=AND(w342, w350, invert w348) -> (w349:bool)
                  }
                }
              }
              n106 = And Array Elements(Boolean array=w177) -> (logical AND=w176:bool)
            }
          }
          n107 = Unbundle By Name(w134) -> ("Pass?"=w137:bool[])
          n108 = Unbundle By Name(w141) -> ("status"=w130:bool)
          n109 = Or(x=w130, y=w128) -> (x .or. y?=w129:bool)
          n110 = Compound Arithmetic op=AND(w131, invert w130) -> (w135:bool)
          n111 = Replace Array Subset(array=w137, new element=w135, index=w126) -> (w136:bool[])
          n112 = Bundle By Name(cluster=w134, "Pass?"=w136) -> (w133:T10)
        }
        n113 = And Array Elements(Boolean array=w100) -> (logical AND=w99:bool)
        n114 = Unbundle By Name(w107) -> ("status"=w90:bool)
        n115 = Or(x=w90, y=w89) -> (x .or. y?=w88:bool)
        n116 = Compound Arithmetic op=AND(w99, invert w90) -> (w101:bool)
      }
      n117 = call "PIM Driver.vi"("Driver Ref (null)"=w62, "PIM Command"=PIM_Command."SET TX OFF") -> ("error out"=w51:errorcluster, "duplicate driver ref"=w54:T12)  [unwired: 3 in, 5 out]
      n118 = Merge Errors(w61, w51) -> (w63:errorcluster)
    }
  }
  "error out" <- w27
  "Pass/Fail" <- w17
  "Measurement Data Out" <- w16
  n119 = Bundle("duplicate driver ref"=w21, "PWM Driver Ref"=w20) -> (→"Driver Refs Out":T28)  [unwired: 1 in]
